vi "Save Data.vi"(8 "error in (no error)":errorcluster, 11 "Pulse Driver in":refnum<class "Pulse Driver.lvclass">) -> (0 "error out":errorcluster, 1 "Finished":bool, 2 "Current read position":i32, 3 "Pulse Driver out":refnum<class "Pulse Driver.lvclass">)   [LabVIEW 2019, in "Pulse Driver.lvclass"]
uses:
  Pulse Driver.lvclass
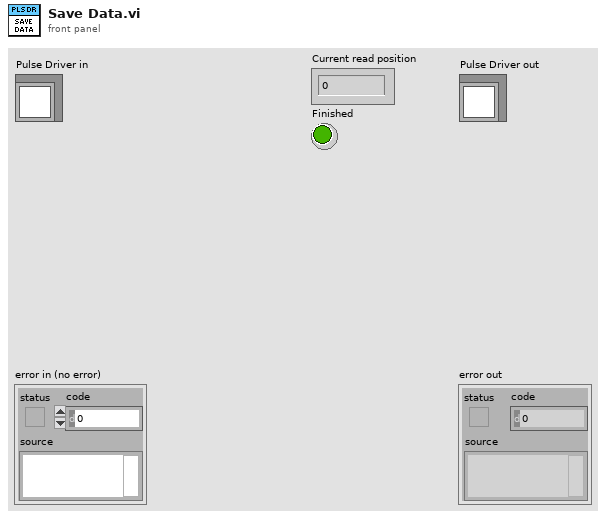
[diagram p1: front panel]
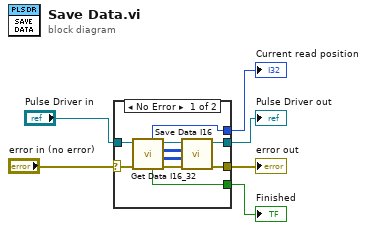
[diagram p0: block diagram]
diagram:
  n1 = case shown="No Error" "error in (no error)" {
    selector: "error in (no error)" -> [w14 w18]
    tunnel: [w13 w18] -> w5
    tunnel: [w11 w17] -> w3
    tunnel: "Pulse Driver in" -> [w12 w17]
    tunnel: [w8 _] -> w2
    tunnel: [w9 _] -> w1
    frame No Error {
      n2 = call-dynamic "Get Data I16_32.vi"("error in (no error)"=w14, "Pulse Driver in"=w12) -> ("error out"=w15:errorcluster, "I32 data out"=w7:i32[][], "I16 data out"=w10:i16[][], "Pulse Driver out"=w16:refnum<class "Pulse Driver.lvclass">, "Finished"=w9:bool, "Current read position"=w8:i32)  [unwired: 4 in]
      n3 = call-dynamic "Save Data I16.vi"("error in (no error)"=w15, "I32 data"=w7, "I16 data"=w10, "Pulse Driver in"=w16) -> ("error out"=w13:errorcluster, "Pulse Driver out"=w11:refnum<class "Pulse Driver.lvclass">)  [unwired: 6 in]
    }
    frame Error {
    }
  }
  "error out" <- w5
  "Pulse Driver out" <- w3
  "Current read position" <- w2
  "Finished" <- w1
